vi "ex_6_zapis_do_pliku.vi"   [LabVIEW 2020]
uses:
  #typedef_Product.ctl
types:
  T1 = typedef "#typedef_Product.ctl" = cluster{"Product Number":i32, "Product Name":string, "Producer":string}
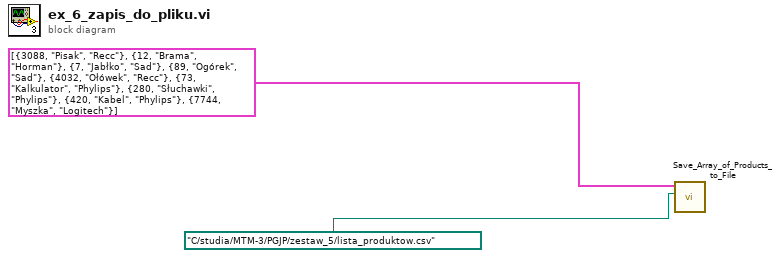
[diagram p0: block diagram]
diagram:
  n1 = call "Save_Array_of_Products_to_File.vi"("Path"=path "C:/studia/MTM-3/PGJP/zestaw_5/lista_produktow.csv", "array of #typedef Products"=T1[] [{"Product Number"=3088, "Product Name"="Pisak", "Producer"="Recc"}, {"Product Number"=12, "Product Name"="Brama", "Producer"="Horman"}, {"Product Number"=7, "Product Name"="Jabłko", "Producer"="Sad"}, {"Product Number"=89, "Product Name"="Ogórek", "Producer"="Sad"}, {"Product Number"=4032, "Product Name"="Ołówek", "Producer"="Recc"}, {"Product Number"=73, "Product Name"="Kalkulator", "Producer"="Phylips"}, {"Product Number"=280, "Product Name"="Słuchawki", "Producer"="Phylips"}, {"Product Number"=420, "Product Name"="Kabel", "Producer"="Phylips"}, {"Product Number"=7744, "Product Name"="Myszka", "Producer"="Logitech"}]) -> ()  [unwired: 10 in]
